vi "util_change_out_write.vi"(7 "references":T1, 8 "error in (no error)":errorcluster, 10 "data":variant, 11 "change":bool) -> (0 "error out":errorcluster)   [LabVIEW 2015, in "lv-recipe-machine.lvlib"]
uses:
  lv-recipe-machine.lvlib
  public/_controls/references.ctl
  public/_controls/input.ctl
  public/_controls/input_command.ctl
  public/_controls/output.ctl
  public/_controls/data.ctl
  public/_controls/configuration.ctl
  public/_controls/recipe_data.ctl
  public/_controls/mode.ctl
  public/_controls/manual_state.ctl
  public/_controls/automatic_state.ctl
  public/_controls/recipe_step.ctl
  <userlib>/antonio-alexander/lv-waitgroup/public/_controls/api_waitgroup.ctl
  public/_controls/change.ctl
  public/_controls/status.ctl
  <userlib>/antonio-alexander/lv-waitgroup/lv-waitgroup.lvlib
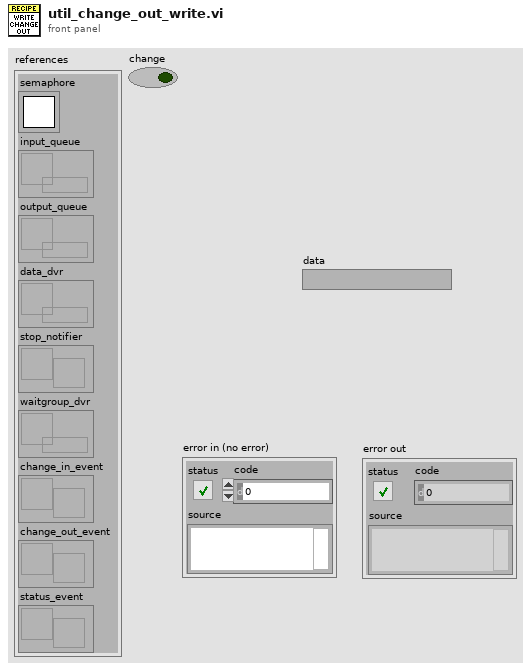
[diagram p1: front panel]
types:
  T1 = typedef "lv-recipe-machine.lvlib/references.ctl" = cluster{"semaphore":T2, "input_queue":refnum<queue>, "output_queue":refnum<queue>, "data_dvr":refnum<data-value>, "stop_notifier":refnum<notifier>, "waitgroup_dvr":refnum<data-value>, "change_in_event":refnum<user-event>, "change_out_event":refnum<user-event>, "status_event":refnum<user-event>}
  T2 = typedef "Semaphore RefNum" = refnum<k1>
  T3 = typedef "lv-recipe-machine.lvlib/change.ctl" = cluster{"data":variant}
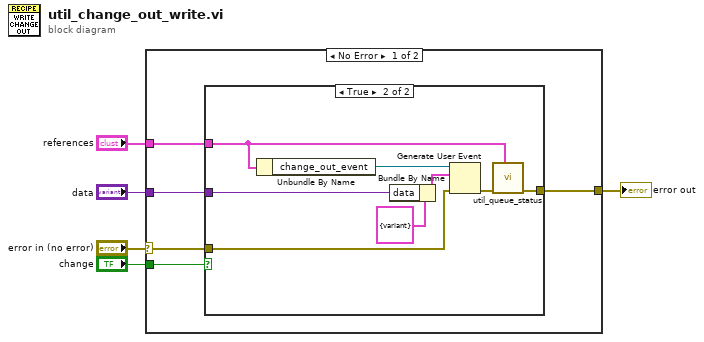
[diagram p0: block diagram]
diagram:
  n1 = case shown="No Error" "error in (no error)" {
    selector: "error in (no error)" -> [w7 w20]
    tunnel: [w8 w20] -> w4
    tunnel: "references" -> [w10 _]
    tunnel: "data" -> [w9 _]
    tunnel: "change" -> [w6 _]
    frame No Error {
      n2 = case shown="True" w6 {
        tunnel: w10 -> [_ w19]
        tunnel: w9 -> [_ w18]
        tunnel: [w11 w17] -> w8
        tunnel: w7 -> [w11 w12]
        frame False {
        }
        frame True {
          n3 = Unbundle By Name(w19) -> ("change_out_event"=w15:refnum<user-event>)
          n4 = Bundle By Name(cluster=T3 {"data"=variant} ("change"), "data"=w18) -> (w13:T3)
          n5 = Generate User Event(user event=w15, event data cluster=w13, error in=w12) -> (error out=w14:errorcluster)  [unwired: 1 in, 1 out]
          n6 = call "util_queue_status.vi"("references"=w19, "error in (no error)"=w14) -> ("error out"=w17:errorcluster)  [unwired: 9 in]
        }
      }
    }
    frame Error {
    }
  }
  "error out" <- w4
